vi "Trigger Pulso (SubVI).vi"(6 "Polarity":u16(ring) items=["Positivo", "Negativo"], 7 "Width":dbl(knob) scale=3.3e-08..10.0, 8 "When":u16(ring) items=["Equal", "NotEqual", "Inside", "Outside"], 9 "Ancho":u16(ring) items=["Polarity", "When", "Width"], 10 "Canal":u16(ring) items=["Canal 1", "Canal 2"], 11 "String de Entrada":string) -> (2 "String de Salida":string, 3 "String de Tipo":string)   [LabVIEW 2019]
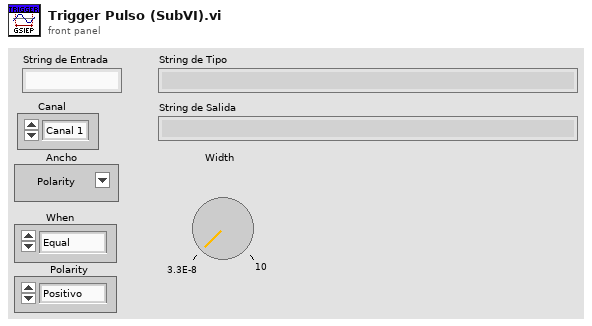
[diagram p1: front panel]
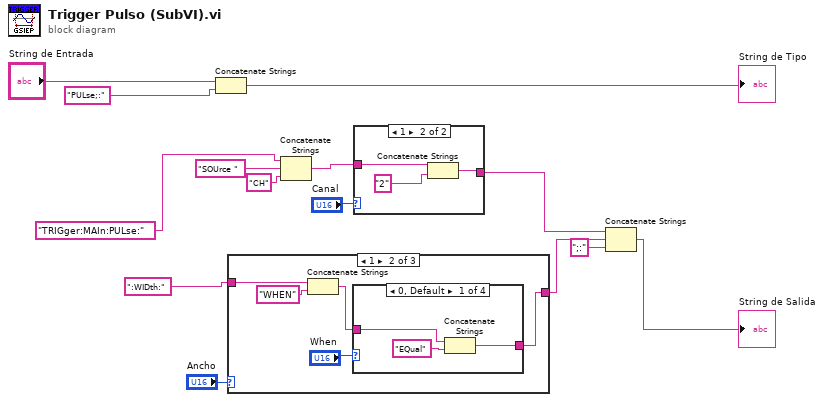
[diagram p0: block diagram]
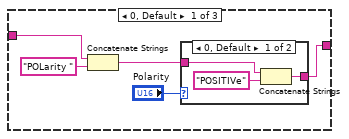
[diagram p2: hidden frame]
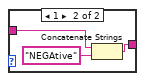
[diagram p3: hidden frame]
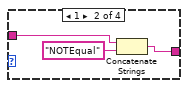
[diagram p4: hidden frame]
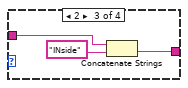
[diagram p5: hidden frame]
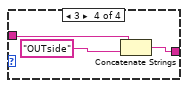
[diagram p6: hidden frame]
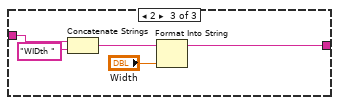
[diagram p7: hidden frame]
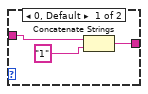
[diagram p8: hidden frame]
diagram:
  n1 = Concatenate Strings("String de Entrada", "PULse;:") -> (→"String de Tipo":string)
  n2 = case shown="1" "Ancho" {
    tunnel: ":WIDth:" -> [w16 w29 w47]
    tunnel: [w15 w26 w43] -> w11
    frame 0, Default {
      n3 = Concatenate Strings(w16, "POLarity ") -> (w17:string)
      n4 = case shown="0, Default" "Polarity" {
        tunnel: w17 -> [w21 w24]
        tunnel: [w20 w23] -> w15
        frame 0, Default {
          n5 = Concatenate Strings(w21, "POSITIVe") -> (w20:string)
        }
        frame 1 {
          n6 = Concatenate Strings(w24, "NEGAtive") -> (w23:string)
        }
      }
    }
    frame 1 {
      n7 = Concatenate Strings(w29, "WHEN") -> (w27:string)
      n8 = case shown="0, Default" "When" {
        tunnel: w27 -> [w32 w35 w38 w41]
        tunnel: [w31 w34 w37 w40] -> w26
        frame 0, Default {
          n9 = Concatenate Strings(w32, "EQual") -> (w31:string)
        }
        frame 1 {
          n10 = Concatenate Strings(w35, "NOTEqual") -> (w34:string)
        }
        frame 2 {
          n11 = Concatenate Strings(w38, "INside") -> (w37:string)
        }
        frame 3 {
          n12 = Concatenate Strings(w41, "OUTside") -> (w40:string)
        }
      }
    }
    frame 2 {
      n13 = Concatenate Strings(w47, "WIDth ") -> (w45:string)
      n14 = Format Into String(initial string=w45, "Width") -> (resulting string=w43:string)  [unwired: 2 in, 1 out]
    }
  }
  n15 = Concatenate Strings("TRIGger:MAIn:PULse:", "SOUrce ", "CH") -> (w5:string)
  n16 = case shown="1" "Canal" {
    tunnel: w5 -> [w49 w52]
    tunnel: [w48 w51] -> w10
    frame 0, Default {
      n17 = Concatenate Strings(w49, "1") -> (w48:string)
    }
    frame 1 {
      n18 = Concatenate Strings(w52, "2") -> (w51:string)
    }
  }
  n19 = Concatenate Strings(w10, w11, ";:") -> (→"String de Salida":string)
